vi "get_shooter_inputs.vi"() -> (3 "Shooter_Inputs":T1)   [LabVIEW 2012]
uses:
  Shooter_inputs.ctl
  <vilib>/Rock Robotics/WPI/CAN/Jaguar/SubVIs/WPI_CANJaguar_StatusSelect.ctl
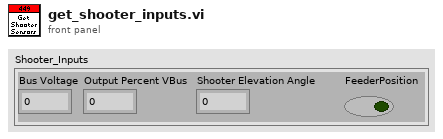
[diagram p1: front panel]
types:
  T1 = typedef "Shooter_inputs.ctl" = cluster{"Bus Voltage":dbl, "Output Percent VBus":dbl, "Shooter Elevation Angle":dbl, "FeederPosition":bool}
  T2 = typedef "WPI_CANJaguar_StatusSelect.ctl" = enum16{"Output Percent VBus", "Output Voltage", "Bus Voltage", "Current", "Temperature", "Position", "Speed", "Limit Switches", "Faults", "Fault Counters", "Power Cycle"}
  T3 = typedef "WPI_MotorControlDeviceRef.ctl" = cluster{"DeviceStatus":errorcluster, "Type":enum16{"PWM", "CAN"}, "PWM":cluster{"Digital Module":T4, "PWM Channel":T5, "DeadBand":T6}, "CAN":cluster{"Device Number":u8, "Control Mode":T7, "Semaphore":T8, "Max Vout":dbl}, "Invert":bool, "TransformRef":T9, "InvTransformRef":T9}
  T4 = typedef "FPGA_TypedefDigitalModule.ctl" = enum16{"Digital Module 1", "Digital Module 2"}
  T5 = typedef "FPGA_DIOPWMChannel.ctl" = enum8{"PWM 1", "PWM 2", "PWM 3", "PWM 4", "PWM 5", "PWM 6", "PWM 7", "PWM 8", "PWM 9", "PWM 10", "Invalid"}
  T6 = typedef "WPI_PWMDeadband.ctl" = cluster{"Name":string, "maxPositivePwm":i32, "minPositivePwm":i32, "centerPwm":i32, "maxNegativePwm":i32, "minNegativePwm":i32, "angularRange":u16}
  T7 = typedef "WPI_CANJaguar_ControlMode.ctl" = enum8{"Percent VBus", "Current", "Speed", "Position", "Voltage"}
  T8 = typedef "Semaphore RefNum" = refnum<k1>
  T9 = typedef "WPI_PWMTransform_ConPane.ctl" = refnum<vi>
  T10 = typedef "WPI_CANJaguar_Status.ctl" = cluster{"Output Percent VBus":dbl, "Output Voltage":dbl, "Bus Voltage":dbl, "Current":dbl, "Temperature":dbl, "Position":dbl, "Speed":dbl, "Limits":cluster{"Forward Limit":bool, "Reverse Limit":bool, "Forward Soft Limit":bool, "Reverse Soft Limit":bool, "Sticky Forward Limit":bool, "Sticky Reverse Limit":bool, "Sticky Forward Soft Limit":bool, "Sticky Reverse Soft Limit":bool}, "Faults":cluster{"Current Fault":bool, "Temperature Fault":bool, "Bus Voltage Fault":bool, "Gate Driver Fault":bool, "Comm Fault":bool}, "Fault Counters":cluster{"Current Faults":u8, "Temperature Faults":u8, "Bus Voltage Faults":u8, "Gate Driver Faults":u8, "Comm Faults":u8, "CAN Status":u8, "CAN RX Errors":u8, "CAN TX Errors":u8}, "Power Cycle":bool}
  T11 = typedef "WPI_DigitalInputDevRef.ctl" = cluster{"DevStatus":errorcluster, "DIO Channel":T12, "Digital Module":T4}
  T12 = typedef "FPGA_DIOChannel.ctl" = enum8{"DIO 1", "DIO 2", "DIO 3", "DIO 4", "DIO 5", "DIO 6", "DIO 7", "DIO 8", "DIO 9", "DIO 10", "DIO 11", "DIO 12", "DIO 13", "DIO 14", "Invalid"}
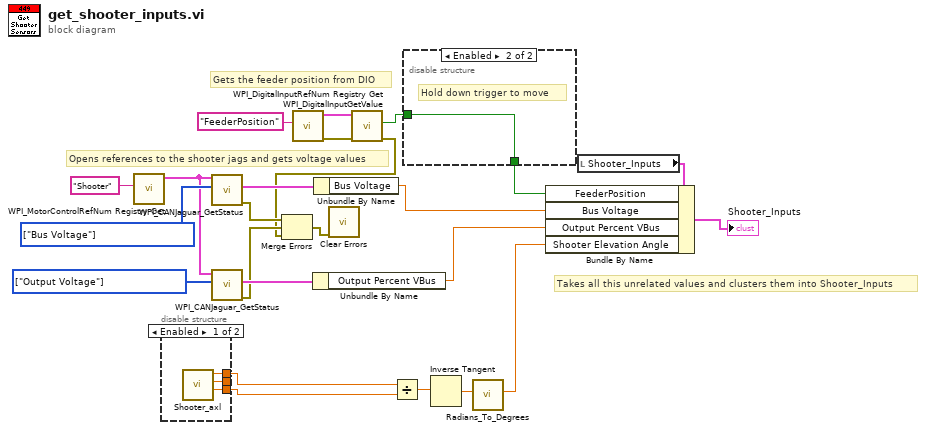
[diagram p0: block diagram]
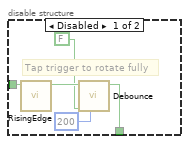
[diagram p3: hidden frame]
diagram:
  w22 = T2[] [enum."Output Voltage"] items=["Output Percent VBus", "Output Voltage", "Bus Voltage", "Current", "Temperature", "Position", "Speed", "Limit Switches", "Faults", "Fault Counters", "Power Cycle"] ("Status Select")
  w23 = T2[] [enum."Bus Voltage"] items=["Output Percent VBus", "Output Voltage", "Bus Voltage", "Current", "Temperature", "Position", "Speed", "Limit Switches", "Faults", "Fault Counters", "Power Cycle"] ("Status Select")
  # "Takes all this unrelated values and clusters them into Shooter_Inputs"
  # "Gets the feeder position from DIO"
  # "Opens references to the shooter jags and gets voltage values"
  n1 = call <vilib>:"WPI_MotorControlRefNum Registry Get.vi"("refnum name"="Shooter") -> ("MotorControlDevRef"=w21:T3)  [unwired: 9 in, 1 out]
  n2 = disable-structure shown="Enabled" {
    disable-tunnel: [w27 _] -> w1
    disable-tunnel: [w26 _] -> _
    disable-tunnel: [w25 _] -> w8
    frame Enabled {
      n3 = call "Shooter_axl.vi"() -> ("Filtered z"=w25:dbl, "Filtered y"=w26:dbl, "Filtered x"=w27:dbl)  [unwired: 9 in]
    }
    frame Disabled {
    }
  }
  n4 = call <vilib>:"WPI_CANJaguar_GetStatus.vi"("Status Select"=w23, "CAN Jaguar Ref"=w21) -> ("error out"=w7:errorcluster, "Status"=w20:T10)  [unwired: 7 in, 1 out]
  n5 = call <vilib>:"WPI_CANJaguar_GetStatus.vi"("Status Select"=w22, "CAN Jaguar Ref"=w21) -> ("error out"=w6:errorcluster, "Status"=w19:T10)  [unwired: 7 in, 1 out]
  n6 = call <vilib>:"WPI_DigitalInputRefNum Registry Get.vi"("refnum name"="FeederPosition") -> ("error out"=w3:errorcluster, "DigitalInputDevRef"=w11:T11)  [unwired: 9 in]
  n7 = Unbundle By Name(w19) -> ("Output Percent VBus"=w17:dbl)
  n8 = Unbundle By Name(w20) -> ("Bus Voltage"=w18:dbl)
  n9 = call <vilib>:"WPI_DigitalInputGetValue.vi"("error in (no error)"=w3, "DigitalInputDevRef"=w11) -> ("error out"=w4:errorcluster, "Value"=w14:bool)  [unwired: 7 in, 1 out]
  n10 = Merge Errors(w7, w6, w4) -> (w5:errorcluster)
  n11 = call <vilib>:"Clear Errors.vi"("error in (no error)"=w5) -> ()  [unwired: 6 in, 1 out]
  n12 = Divide(x=w1, y=w8) -> (x/y=w9:dbl)
  n13 = disable-structure shown="Enabled" {
    disable-tunnel: w14 -> [w32 w33]
    disable-tunnel: [w30 w33] -> w13
    frame Disabled {
      # "Tap trigger to rotate fully"
      n14 = call "RisingEdge.vi"("BooleanIn"=w32) -> ("BooleanOut"=w31:bool)  [unwired: 10 in]
      n15 = call "Debounce.vi"("Time Threshold"=u32 200, "Default Value"=FALSE, "Boolean In"=w31) -> ("Boolean Out"=w30:bool)  [unwired: 8 in]
    }
    frame Enabled {
      # "Hold down trigger to move"
    }
  }
  n16 = Inverse Tangent(1:w9) -> (0:w10:dbl)
  n17 = call "Radians_To_Degrees.vi"("Radians"=w10) -> ("Degrees"=w2:dbl)  [unwired: 10 in]
  n18 = local read "Shooter_Inputs"() -> (w15:T1)
  n19 = Bundle By Name(cluster=w15, "FeederPosition"=w13, "Bus Voltage"=w18, "Output Percent VBus"=w17, "Shooter Elevation Angle"=w2) -> (→"Shooter_Inputs":T1)
